vi "Get Adjascent Bool.vi"(9 "column":i32, 10 "row":i32, 11 "Array in":bool[][](array[boolean])) -> (3 "Array out":bool[](array[boolean]))   [LabVIEW 2019, in "Day 9.lvlib"]
uses:
  Day 9.lvlib
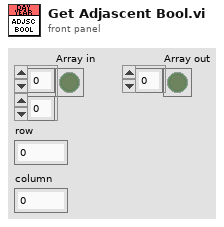
[diagram p1: front panel]
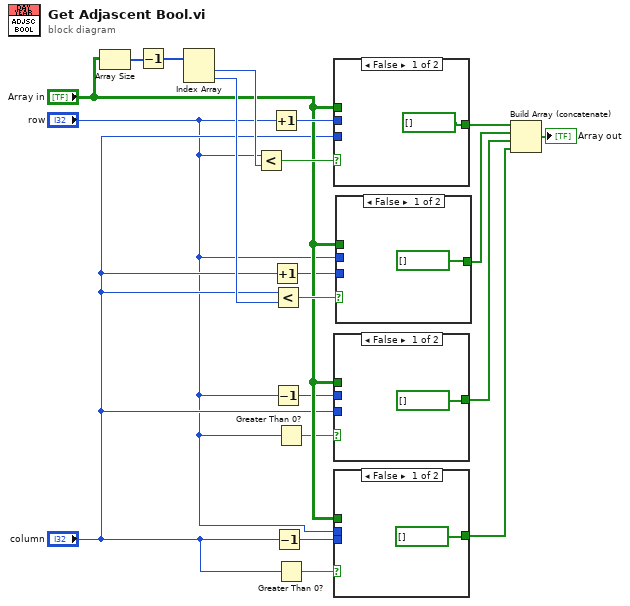
[diagram p0: block diagram]
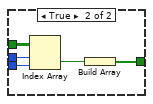
[diagram p2: hidden frame]
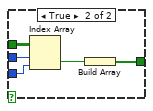
[diagram p3: hidden frame]
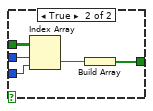
[diagram p4: hidden frame]
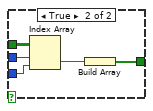
[diagram p5: hidden frame]
diagram:
  n1 = Array Size(array="Array in") -> (size(s)=w2:i32[])
  n2 = Decrement(x=w2) -> (x-1=w1:i32[])
  n3 = Index Array(array=w1) -> (element #1=w19:i32, element #2=w17:i32)  [unwired: 2 in]
  n4 = Less?(x="row", y=w19) -> (x < y?=w18:bool)
  n5 = Increment(x="row") -> (x+1=w20:i32)
  n6 = Increment(x="column") -> (x+1=w14:i32)
  n7 = Less?(x="column", y=w17) -> (x < y?=w16:bool)
  n8 = Decrement(x="row") -> (x-1=w12:i32)
  n9 = Decrement(x="column") -> (x-1=w10:i32)
  n10 = Greater Than 0?(x="row") -> (x > 0?=w13:bool)
  n11 = Greater Than 0?(x="column") -> (x > 0?=w9:bool)
  n12 = case shown="False" w18 {
    tunnel: w20 -> [_ w26]
    tunnel: "Array in" -> [_ w25]
    tunnel: "column" -> [_ w24]
    tunnel: [bool[] [] w22] -> w7
    frame False {
    }
    frame True {
      n13 = Index Array(array=w25, index (row)=w26, index (col)=w24) -> (element=w23:bool)
      n14 = Build Array(w23) -> (w22:bool[])
    }
  }
  n15 = case shown="False" w13 {
    tunnel: w12 -> [_ w32]
    tunnel: "Array in" -> [_ w31]
    tunnel: "column" -> [_ w30]
    tunnel: [bool[] [] w28] -> w5
    frame False {
    }
    frame True {
      n16 = Index Array(array=w31, index (row)=w32, index (col)=w30) -> (element=w29:bool)
      n17 = Build Array(w29) -> (w28:bool[])
    }
  }
  n18 = case shown="False" w9 {
    tunnel: "row" -> [_ w38]
    tunnel: "Array in" -> [_ w37]
    tunnel: w10 -> [_ w36]
    tunnel: [bool[] [] w34] -> w4
    frame False {
    }
    frame True {
      n19 = Index Array(array=w37, index (row)=w38, index (col)=w36) -> (element=w35:bool)
      n20 = Build Array(w35) -> (w34:bool[])
    }
  }
  n21 = case shown="False" w16 {
    tunnel: "row" -> [_ w44]
    tunnel: "Array in" -> [_ w43]
    tunnel: w14 -> [_ w42]
    tunnel: [bool[] [] w40] -> w6
    frame False {
    }
    frame True {
      n22 = Index Array(array=w43, index (row)=w44, index (col)=w42) -> (element=w41:bool)
      n23 = Build Array(w41) -> (w40:bool[])
    }
  }
  n24 = Build Array (concatenate)(w7, w6, w5, w4) -> (→"Array out":bool[])
